vi "Initialize.vi"(0 "VISA Resource Name":refnum<visa-resource-name>="GPIB0::9::INSTR", 5 "ID Query (T: Check)":bool=TRUE, 7 "Reset (T: Reset)":bool=TRUE, 9 "Serial Port Configuration":T1={"Timeout Value (10000)"=10000, "Baud Rate (57600)"=enum."57600", "Flow Control (1:XON/XOFF)"=enum."XON / XOFF"}, 11 "error in (no error)":errorcluster) -> (4 "VISA Resource Name Out":refnum<visa-resource-name>, 15 "error out":errorcluster)   [LabVIEW 2018, in "Agilent 34970.lvlib"]
doc: "This VI passes the addressing information in the instrument decriptor to the Instr Open VI and returns the instrument ID. You can optionally reset the instrument by setting the front panel reset control. You must run this VI before using any of the instrument driver VIs for this instrument.\n\nSupported Modules: \n34901A 20-Channel Armature Multiplexer\n34902A 16-Channel Reed Multiplexer\n34903A 20-Channel Actuator / General-Purpose Switch\n34904A 4x8 Two-Wire Matrix Switch\n34905/6A Dual 4-Channel RF Multiplexers\n34907A Multifunction Module\n34908A 40-Channel Single-Ended Multiplexer"
uses:
  Agilent 34970.lvlib
panel:
  # "(c) 2005-2010 National Instruments.  ALL RIGHTS RESERVED."
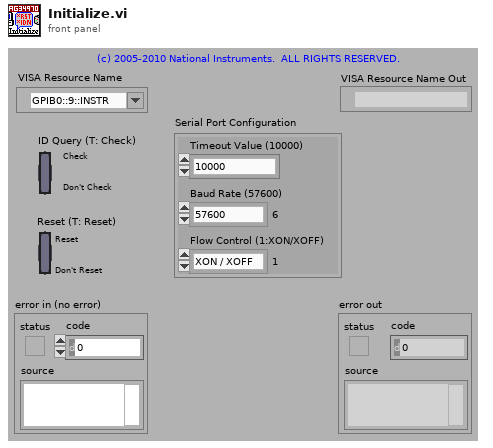
[diagram p1: front panel]
types:
  T1 = cluster{"Timeout Value (10000)":u32, "Baud Rate (57600)":enum16{"1200", "2400", "4800", "9600", "19200", "38400", "57600", "115200"}, "Flow Control (1:XON/XOFF)":enum16{"None", "XON / XOFF", "RTS / CTS", "DTR / DSR"}}
  T2 = enum16{"1200", "2400", "4800", "9600", "19200", "38400", "57600", "115200"}
  T3 = enum16{"None", "XON / XOFF", "RTS / CTS", "DTR / DSR"}
  T4 = cluster{"Status":bool, "Code":i32, "Source (VI Name)":string}
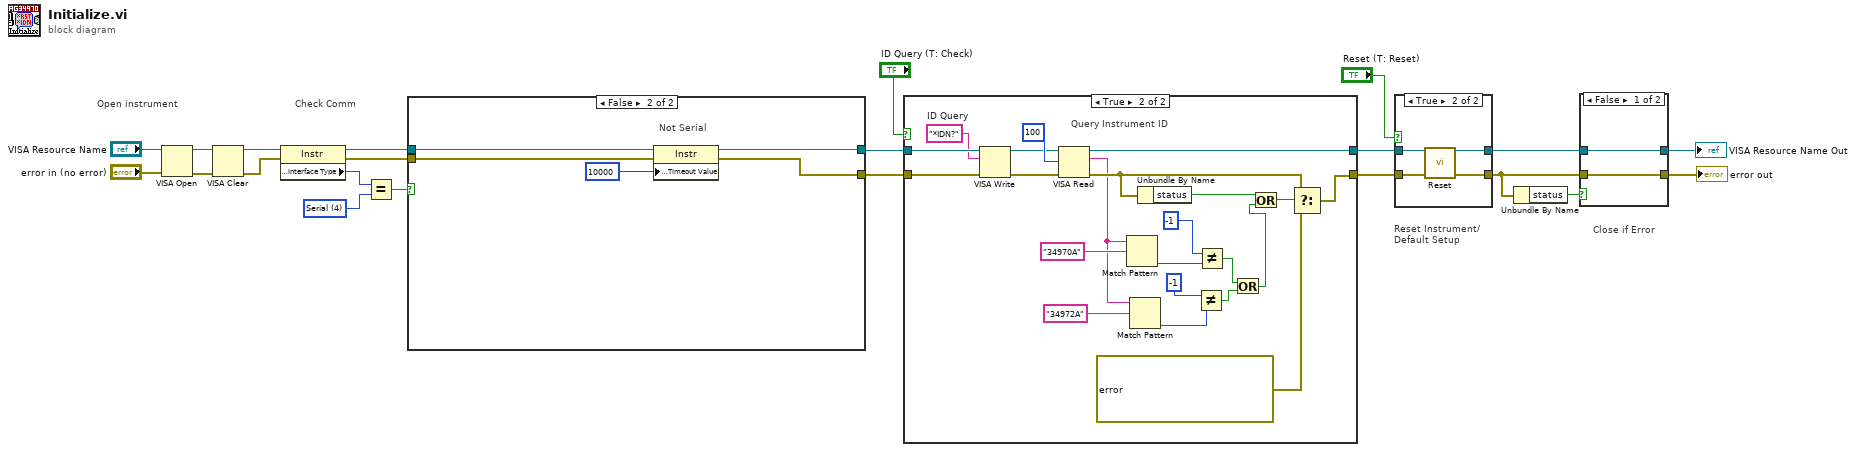
[diagram p0: block diagram]
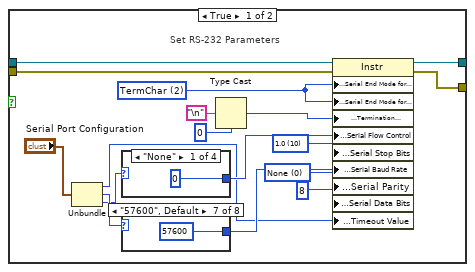
[diagram p2: hidden frame]
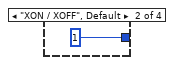
[diagram p3: hidden frame]
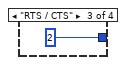
[diagram p4: hidden frame]
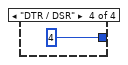
[diagram p5: hidden frame]
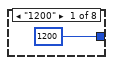
[diagram p6: hidden frame]
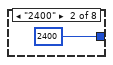
[diagram p7: hidden frame]
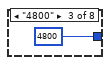
[diagram p8: hidden frame]
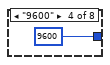
[diagram p9: hidden frame]
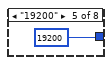
[diagram p10: hidden frame]
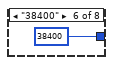
[diagram p11: hidden frame]
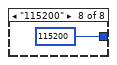
[diagram p12: hidden frame]
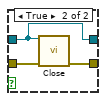
[diagram p13: hidden frame]
diagram:
  w15 = u16 4 items=["GPIB"=1, "VXI"=2, "GPIB-VXI"=3, "Serial"=4, "PXI"=5] ("Interface Information:Interface Type")
  # "Check Comm"
  # "Close if Error"
  # "Reset Instrument/\nDefault Setup"
  # "Open instrument"
  n1 = VISA Open(error in (no error)="error in (no error)", VISA resource name="VISA Resource Name") -> (VISA resource name=w5:refnum<visa-resource-name>, error out=w4:errorcluster)  [unwired: 3 in]
  n2 = VISA Clear(VISA resource name=w5, error in (no error)=w4) -> (VISA resource name out=w3:refnum<visa-resource-name>, error out=w2:errorcluster)
  n3 = property on="Property Node" class="Instr"(reference=w3, error in=w2) -> (reference out=w17:refnum<visa-resource-name>, error out=w16:errorcluster, "Interface Information:Interface Type"=w1:u16)
  n4 = Equal?(x=w1, y=w15) -> (x = y?=w14:bool)
  n5 = case shown="False" w14 {
    tunnel: [w28 w54] -> w13
    tunnel: w17 -> [w39 w56]
    tunnel: [w27 w52] -> w12
    tunnel: w16 -> [w38 w55]
    frame True {
      w30 = u16 0 items=["None", "Odd", "Even", "Mark", "Space"] ("Serial Settings:Serial Parity")
      w31 = u16 10 items=["1.0"=10, "1.5"=15, "2.0"=20] ("Serial Settings:Serial Stop Bits")
      w35 = u16 2 items=["None", "LastBit", "TermChar"] ("Serial Settings:Serial End Mode for Reads")
      # "Set RS-232 Parameters"
      n6 = Unbundle("Serial Port Configuration") -> ("Timeout Value (10000)"=w23:u32, "Baud Rate (57600)"=w25:T2, "Flow Control (1:XON/XOFF)"=w24:T3)
      n7 = case shown="\"None\"" w24 {
        tunnel: [u16 0 u16 1 u16 2 u16 4] -> w36
        frame "None" {
        }
        frame "XON / XOFF", Default {
        }
        frame "RTS / CTS" {
        }
        frame "DTR / DSR" {
        }
      }
      n8 = case shown="\"57600\", Default" w25 {
        tunnel: [u32 1200 u32 2400 u32 4800 u32 9600 u32 19200 u32 38400 u32 57600 u32 115200] -> w37
        frame "1200" {
        }
        frame "2400" {
        }
        frame "4800" {
        }
        frame "9600" {
        }
        frame "19200" {
        }
        frame "38400" {
        }
        frame "57600", Default {
        }
        frame "115200" {
        }
      }
      n9 = Type Cast(type=u8 0, x="\n" ("Line Feed Constant")) -> (*(type *) &x=w32:u8)
      n10 = property on="Property Node" class="Instr"(reference=w39, error in=w38, "Serial Settings:Serial End Mode for Reads"=w35, "Serial Settings:Serial End Mode for Writes"=w35, "Message Based Settings:Termination Character"=w32, "Serial Settings:Serial Flow Control"=w36, "Serial Settings:Serial Stop Bits"=w31, "Serial Settings:Serial Baud Rate"=w37, "Serial Settings:Serial Parity"=w30, "Serial Settings:Serial Data Bits"=u16 8, "General Settings:Timeout Value"=w23) -> (reference out=w28:refnum<visa-resource-name>, error out=w27:errorcluster)
    }
    frame False {
      # "Not Serial"
      n11 = property on="Property Node" class="Instr"(reference=w56, error in=w55, "General Settings:Timeout Value"=u32 10000 ("Tmo Value")) -> (reference out=w54:refnum<visa-resource-name>, error out=w52:errorcluster)
    }
  }
  n12 = case shown="True" "ID Query (T: Check)" {
    tunnel: [w57 w80] -> w21
    tunnel: [w58 w77] -> w22
    tunnel: w13 -> [w58 w78]
    tunnel: w12 -> [w57 w79]
    frame False {
    }
    frame True {
      w67 = "*IDN?"  # ID Query
      # "Query Instrument ID"
      n13 = VISA Write(VISA resource name=w78, write buffer=w67, error in (no error)=w79) -> (VISA resource name out=w69:refnum<visa-resource-name>, error out=w71:errorcluster)  [unwired: 1 out]
      n14 = VISA Read(VISA resource name=w69, byte count=u32 100, error in (no error)=w71) -> (VISA resource name out=w77:refnum<visa-resource-name>, read buffer=w62:string, error out=w70:errorcluster)  [unwired: 1 out]
      n15 = Match Pattern(string=w62, regular expression="34970A") -> (offset past match=w75:i32)  [unwired: 1 in, 3 out]
      n16 = Match Pattern(string=w62, regular expression="34972A") -> (offset past match=w65:i32)  [unwired: 1 in, 3 out]
      n17 = Unbundle By Name(w70) -> ("status"=w68:bool)
      n18 = Not Equal?(x=-1, y=w65) -> (x != y?=w61:bool)
      n19 = Not Equal?(x=-1, y=w75) -> (x != y?=w60:bool)
      n20 = Or(x=w60, y=w61) -> (x .or. y?=w59:bool)
      n21 = Or(x=w68, y=w59) -> (x .or. y?=w72:bool)
      n22 = Select(t=w70, s=w72, f=T4 {"Status"=TRUE, "Code"=-1074003951, "Source (VI Name)"="<ERR> PREFIX Initialize\nThe ID Query failed.  This may mean that you selected the wrong instrument or your instrument did not respond.  You may also be using a model that is not officially supported by this driver.  If you are sure that you have selected the correct instrument and it is responding, try disabling the ID Query."}) -> (s? t:f=w80:T4)
    }
  }
  n23 = case shown="True" "Reset (T: Reset)" {
    tunnel: w21 -> [w81 w83]
    tunnel: [w81 w86] -> w19
    tunnel: w22 -> [w82 w84]
    tunnel: [w82 w85] -> w18
    frame False {
    }
    frame True {
      n24 = call "Reset.vi"("VISA Resource Name"=w84, "error in (no error)"=w83) -> ("VISA Resource Name Out"=w85:refnum<visa-resource-name>, "error out"=w86:errorcluster)  [unwired: 12 in]
    }
  }
  n25 = Unbundle By Name(w19) -> ("status"=w20:bool)
  n26 = case shown="False" w20 {
    tunnel: w18 -> [w87 w89]
    tunnel: w19 -> [w88 w91]
    tunnel: [w88 w90] -> w10
    tunnel: [w87 w89] -> w7
    frame False {
    }
    frame True {
      n27 = call "Close.vi"("VISA Resource Name"=w89, "error in (no error)"=w91) -> ("error out"=w90:errorcluster)  [unwired: 13 in]
    }
  }
  "error out" <- w10
  "VISA Resource Name Out" <- w7
